vi "Focus Fiducial.vi"(8 "error in":errorcluster, 10 "Component In":T1, 11 "Gantry In":refnum<k24>) -> (0 "error out":errorcluster, 2 "Component Out":T1, 3 "Gantry Out":refnum<k24>)   [LabVIEW 2021, in "Component Tray.lvclass"]
uses:
  Component/Component Tray.lvclass
  C:/Program Files (x86)/Aerotech/A3200/LabVIEW/2010/Bin/Aerotech.A3200.dll
  Program Files (x86)/Aerotech/A3200/LabVIEW/2010/Bin/Aerotech.A3200.dll
  Component/Find Component.ctl
  Controller/Camera/Machine Vision.ctl
  Component/Component Tray.lvclass/Component Tray.ctl
  Controller/Camera/Camera.lvclass
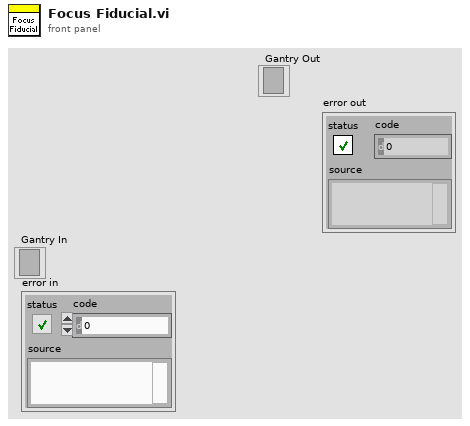
[diagram p1: front panel]
types:
  T1 = typedef "Component Tray.lvclass/Find Component.ctl" = cluster{"New Fiducials":dbl[], "Past Fiducials":dbl[][], "XYZTheta":dbl[], "Fiducials Path":path, "Position":i32, "CH1 Location":dbl[], "Sensor ID Location":dbl[], "initial rotation":dbl[], "CH2 location":dbl[], "max std variation":dbl, "max strength":dbl, "CH2 pattern matching":T2, "Fiducial Circle":T2, "Get Edge":T2, "Pos multiplier":dbl, "time to wait":u32, "fiducial to edge":dbl, "Protomodule?":bool, "Assembly Type":string, "CH1 to CH2":dbl, "Tray Number":string, "fiducial radius":dbl, "4 fiducials?":bool, "CH1 check":T2, "Edge Scan":T2, "CH1 pattern matching":T2, "Sensor Thickness":dbl, "Previous Avgs":dbl[][], "avg value count":dbl[]}
  T2 = typedef "Camera.lvclass/Machine Vision.ctl" = enum16{"None", "Assembly Tray Circle", "Assembly Tray Fiducial", "Partial Hexaboard", "sensor edge init", "HB edge init", "sensor edge pos1", "sensor edge pos2", "HB edge pos1", "HB edge pos2", "Sensor CH1-2", "HB CH1", "HB CH2", "V3 Sensor Circle", "Hexaboard Circle", "sensor CH1 check", "HB CH1 check ", "sensor ID"}
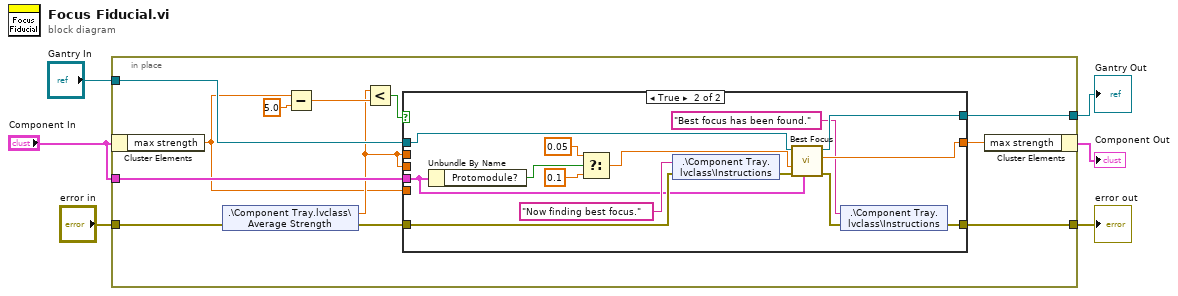
[diagram p0: block diagram]
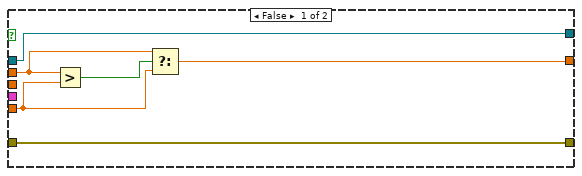
[diagram p2: hidden frame]
diagram:
  n1 = in-place {
    in-place-border: "Gantry In" -> [w18]
    in-place-border: "error in" -> [w13]
    in-place-border: [w17] -> w4
    in-place-border: [w16] -> w3
    in-place-border: "Component In" -> [w9]
    n2 = in-place-cluster #1("Component In") -> ("max strength"=w7:dbl)
    n3 = shared-variable ".\\Component Tray.lvclass\\Average Strength"(error in=w13) -> (w8:dbl, error out=w12:errorcluster)
    n4 = Subtract(x=w7, y=5.0) -> (x-y=w14:dbl)
    n5 = Less?(x=w8, y=w14) -> (x < y?=w11:bool)
    n6 = case shown="True" w11 {
      tunnel: w18 -> [w20 w38]
      tunnel: [w20 w36] -> w17
      tunnel: [w19 w31] -> w16
      tunnel: w12 -> [w19 w37]
      tunnel: w8 -> [w23 _]
      tunnel: w7 -> [w22 _]
      tunnel: [w21 w35] -> w10
      tunnel: w9 -> [_ w29]
      tunnel: w8 -> [_ _]
      frame False {
        n7 = Greater?(x=w23, y=w22) -> (0:w24:bool)
        n8 = Select(t=w23, s=w24, f=w22) -> (s? t:f=w21:dbl)
      }
      frame True {
        n9 = Unbundle By Name(w29) -> ("Protomodule?"=w28:bool)
        n10 = Select(t=0.05 ("Inc by"), s=w28, f=0.1 ("Inc by")) -> (s? t:f=w27:dbl)
        n11 = shared-variable ".\\Component Tray.lvclass\\Instructions"("Now finding best focus." ("Instructions"), error in=w37) -> (error out=w34:errorcluster)
        n12 = call "Best Focus.vi"("Component"=w29, "error in (no error)"=w34, "Inc by"=w27, "Gantry In"=w38) -> ("error out"=w32:errorcluster, "max value"=w35:dbl, "Gantry Out"=w36:refnum<k24>)  [unwired: 4 in, 1 out]
        n13 = shared-variable ".\\Component Tray.lvclass\\Instructions"("Best focus has been found." ("Instructions"), error in=w32) -> (error out=w31:errorcluster)
      }
    }
    n14 = in-place-cluster #1("max strength"=w10) -> (→"Component Out":T1)
  }
  "Gantry Out" <- w4
  "error out" <- w3
